vi "Queue Basics.vi"() -> ()   [LabVIEW 2010]
doc: "Demonstrates general use of Obtain Queue, queues and the effects different settings have on queue behavior. It uses a queue to pass data between an Enqueue loop (producing data) and a Dequeue loop (consuming data). If both loops run at the same speed, the queue does not fill up.\n\nWhen the Enqueue loop runs fast and the Dequeue loop runs slow, the queue quickly fills up and the Enqueue loop must wait for the Dequeue loop to remove elements. If the Enqueue loop runs slow and the Dequeue loop runs fast, the queue is quickly emptied and the Dequeue loop must wait for the Enqueue loop to insert elements."
panel:
  out "Last Element Removed":dbl format="%0.2f"
  in  "Enqueue Speed":bool
  in  "Dequeue Speed":bool
  out "Waveform Chart":cluster{"Last Element Inserted":dbl, dbl}(graph)
  out "Elements in Queue":i32(slide) scale=0.0..5.0 scale format="%0.0f"
  in  "stop":bool
  in  "Queue Size":i32=50
  out "Last Element Inserted":dbl format="%0.2f"
  # "Instructions:\n1. Select the Queue size you would like to use.\n2. Run VI.\n3. Adjust the Enqueue Speed and Dequeue\n    Speed controls to see the Elements\n    in Queue indicator and Waveform\n    chart plots change."
  # "Fast (100ms)\n\nSlow (500ms)"
  # "Fast (100ms)\n\nSlow (500ms)"
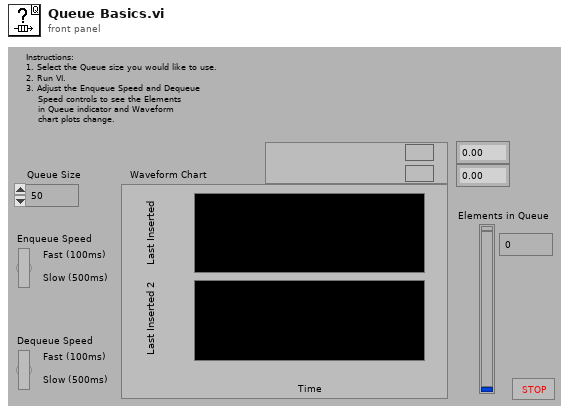
[diagram p1: front panel]
types:
  T1 = cluster{"Last Element Inserted":dbl, "Last Element Removed":dbl}
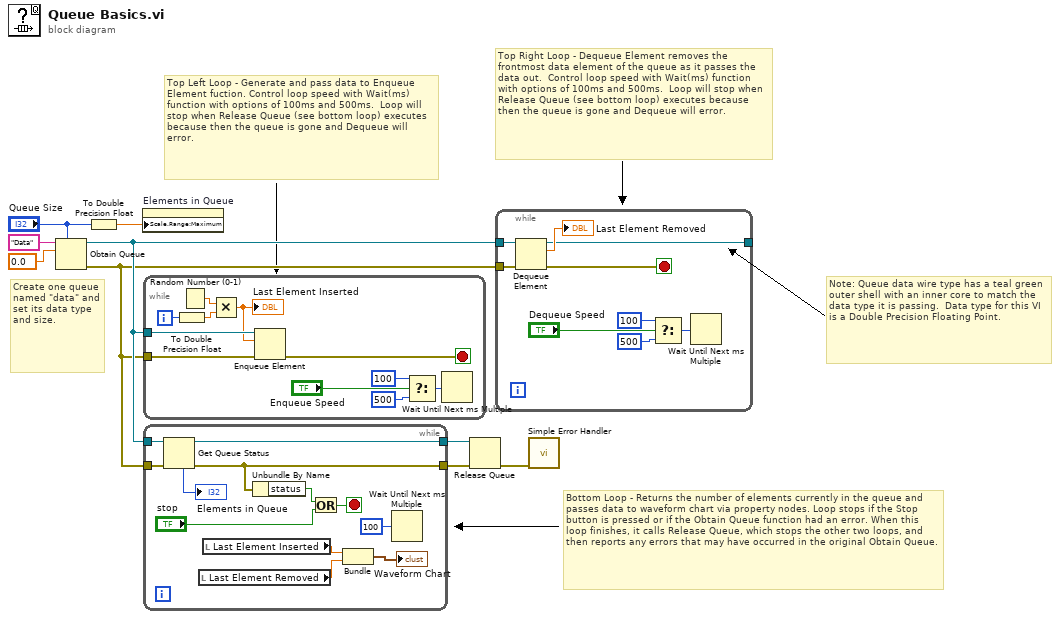
[diagram p0: block diagram]
diagram:
  # "Top Right Loop - Dequeue Element removes the frontmost data element of the queue as it passes the data out.  Control loop speed with Wait(ms) function with options of 100ms and 500ms.  Loop will stop when Release Queue (see bottom loop) executes because then the queue is gone and Dequeue will error."
  # "Note: Queue data wire type has a teal green outer shell with an inner core to match the data type it is passing.  Data type for this VI is a Double Precision Floating Point."
  # "Bottom Loop - Returns the number of elements currently in the queue and passes data to waveform chart via property nodes. Loop stops if the Stop button is pressed or if the Obtain Queue function had an error. When this loop finishes, it calls Release Queue, which stops the other two loops, and then reports any errors that may have occurred in the original Obtain Queue."
  # "Top Left Loop - Generate and pass data to Enqueue Element fuction. Control loop speed with Wait(ms) function with options of 100ms and 500ms.  Loop will stop when Release Queue (see bottom loop) executes because then the queue is gone and Dequeue will error."
  # "Create one queue named \"data\" and set its data type and size."
  n1 = Obtain Queue(max queue size (-1, unlimited)="Queue Size", name (unnamed)="Data", element data type=0.0) -> (queue out=w9:refnum<queue>, error out=w4:errorcluster)  [unwired: 2 in, 1 out]
  n2 = To Double Precision Float(number="Queue Size") -> (double precision float=w8:dbl)
  n3 = property on="Elements in Queue" class="Slide (strict)"("Scale.Range:Maximum"=w8) -> ()  [unwired: 2 in, 2 out]
  n4 = while {
    tunnel: w9 -> [w20]
    tunnel: w4 -> [w11]
    i -> [w18]
    stop <- w10 stop-if-true
    n5 = To Double Precision Float(number=w18) -> (double precision float=w17:dbl)
    n6 = Random Number (0-1)() -> (number: 0 to 1=w19:dbl)
    n7 = Multiply(x=w19, y=w17) -> (x*y=w16:dbl)
    "Last Element Inserted" <- w16
    n8 = Enqueue Element(queue=w20, element=w16, error in (no error)=w11) -> (error out=w10:errorcluster)  [unwired: 3 out]
    n9 = Select(t=u32 100, s="Enqueue Speed", f=u32 500) -> (s? t:f=w12:u32)
    n10 = Wait Until Next ms Multiple(millisecond multiple=w12) -> ()  [unwired: 1 out]
  }
  n11 = while {
    tunnel: w9 -> [w32]
    tunnel: [w21] -> w3
    tunnel: w4 -> [w25]
    tunnel: [w22] -> w2
    stop <- w28 stop-if-true
    n12 = Get Queue Status(queue=w32, error in (no error)=w25) -> (queue out=w22:refnum<queue>, error out=w21:errorcluster, # elements in queue=→"Elements in Queue":i32)  [unwired: 6 out]
    n13 = local read "Last Element Removed"() -> (w23:dbl)
    n14 = local read "Last Element Inserted"() -> (w24:dbl)
    n15 = Unbundle By Name(w21) -> ("status"=w27:bool)
    n16 = Or(x=w27, y="stop") -> (x .or. y?=w28:bool)
    n17 = Bundle("Last Element Inserted"=w24, "Last Element Removed"=w23) -> (→"Waveform Chart":T1)  [unwired: 1 out]
    n18 = Wait Until Next ms Multiple(millisecond multiple=u32 100 ("milliseconds to wait")) -> ()  [unwired: 1 out]
  }
  n19 = Release Queue(queue=w2, error in (no error)=w3) -> (error out=w1:errorcluster)  [unwired: 3 out]
  n20 = while {
    tunnel: w9 -> [w41]
    tunnel: [w35] -> _
    tunnel: w4 -> [w34]
    stop <- w33 stop-if-true
    n21 = Dequeue Element(queue=w41, error in (no error)=w34) -> (queue out=w35:refnum<queue>, element=→"Last Element Removed":dbl, error out=w33:errorcluster)  [unwired: 2 out]
    n22 = Select(t=u32 100, s="Dequeue Speed", f=u32 500) -> (s? t:f=w37:u32)
    n23 = Wait Until Next ms Multiple(millisecond multiple=w37) -> ()  [unwired: 1 out]
  }
  n24 = call <vilib>:"Simple Error Handler.vi"("error in (no error)"=w1) -> ()  [unwired: 1 in, 8 out]
